vi "Current Position Read.vi"(4 "error in (no error)":errorcluster, 6 "Container State":T2, 7 "Display State In":T1) -> (0 "error out":errorcluster, 2 "Value":i32, 3 "Display State Out":T1)   [LabVIEW 2012, in "Vector Function Generator.xctl"]
doc: "Reads the location of the current position marker"
uses:
  Vector Function Generator.xctl
  <vilib>/_xctls/Container State.ctl
  Vector State.ctl
  <vilib>/_xctls/XControlSupport.lvlib
panel:
  # "Replace the Value Indicator below with an Indicator of desired type.\nDo not remove this Indicator or the others from the connector pane. \nDo not change the connector pane pattern.\nThe Value Indicator should always be the second terminal from top on the output side in the connector pane."
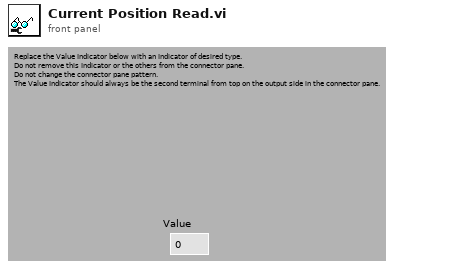
[diagram p1: front panel]
types:
  T1 = typedef "Vector Function Generator.xctl/Vector State.ctl" = cluster{"Current Position":i32, "Show Current Position":bool, "Mode (F=Polar)":bool, "digits":i32, "sf(F) or dp ?":bool, "Units":string}
  T2 = typedef "XControlSupport.lvlib/Container State.ctl" = cluster{"Indicator?":bool, "Run Mode?":bool, " Refnum":refnum<vi>}
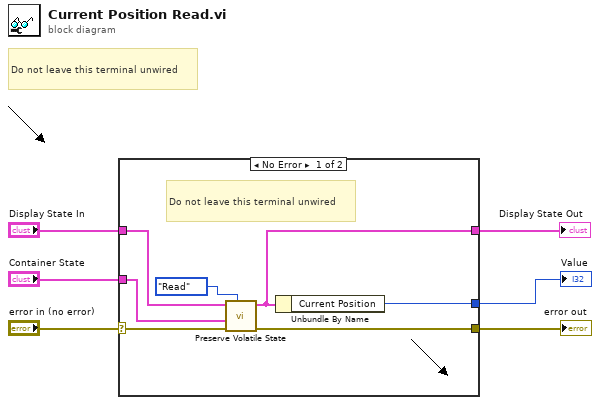
[diagram p0: block diagram]
diagram:
  # "Do not leave this terminal unwired"
  n1 = case shown="No Error" "error in (no error)" {
    selector: "error in (no error)" -> [w10 w15]
    tunnel: [w13 _] -> w3
    tunnel: "Display State In" -> [w12 w14]
    tunnel: "Container State" -> [w11 _]
    tunnel: [w9 w15] -> w2
    tunnel: [w8 w14] -> w4
    frame No Error {
      # "Do not leave this terminal unwired"
      n2 = call "Preserve Volatile State.vi"("Operation In"=enum16{"Read", "Write", "Update From Data"}."Read" ("Operation"), "Error In (no Error) In"=w10, "Container State In"=w11, "Waveform State In"=w12) -> ("Error Out"=w9:errorcluster, "Waveform State Out"=w8:T1)  [unwired: 1 in, 5 out]
      n3 = Unbundle By Name(w8) -> ("Current Position"=w13:i32)
    }
    frame Error {
    }
  }
  "error out" <- w2
  "Value" <- w3
  "Display State Out" <- w4
